vi "GSP_Wavelength_GenerateScript.vi"(0 "Current Grating":dbl, 1 "Current Camera":dbl, 2 "Target Grating":dbl, 3 "Target Camera":dbl, 4 "Move type":T1 items=["Both", "Grating Only", "Camera Only"]) -> (5 "Script":cluster{string, string}[](array[cluster]), 6 "AllowMove?":bool)   [LabVIEW 2015]
uses:
  movetypes.ctl
  wavelength_parameters.ctl
  GSCS Scripting/Utils/GSP_Wavelength_Global.vi
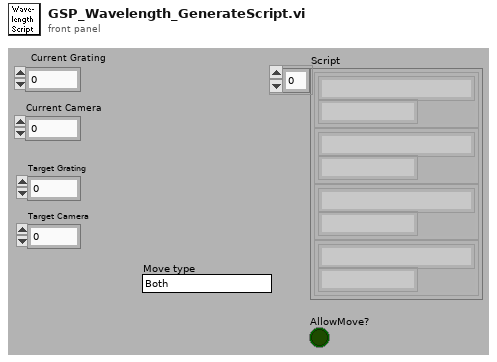
[diagram p1: front panel]
types:
  T1 = typedef "movetypes.ctl" = u16
  T2 = typedef "wavelength_parameters.ctl" = cluster{"Camera Angle":dbl, "Grating  Angle":dbl, "Move type":T1}
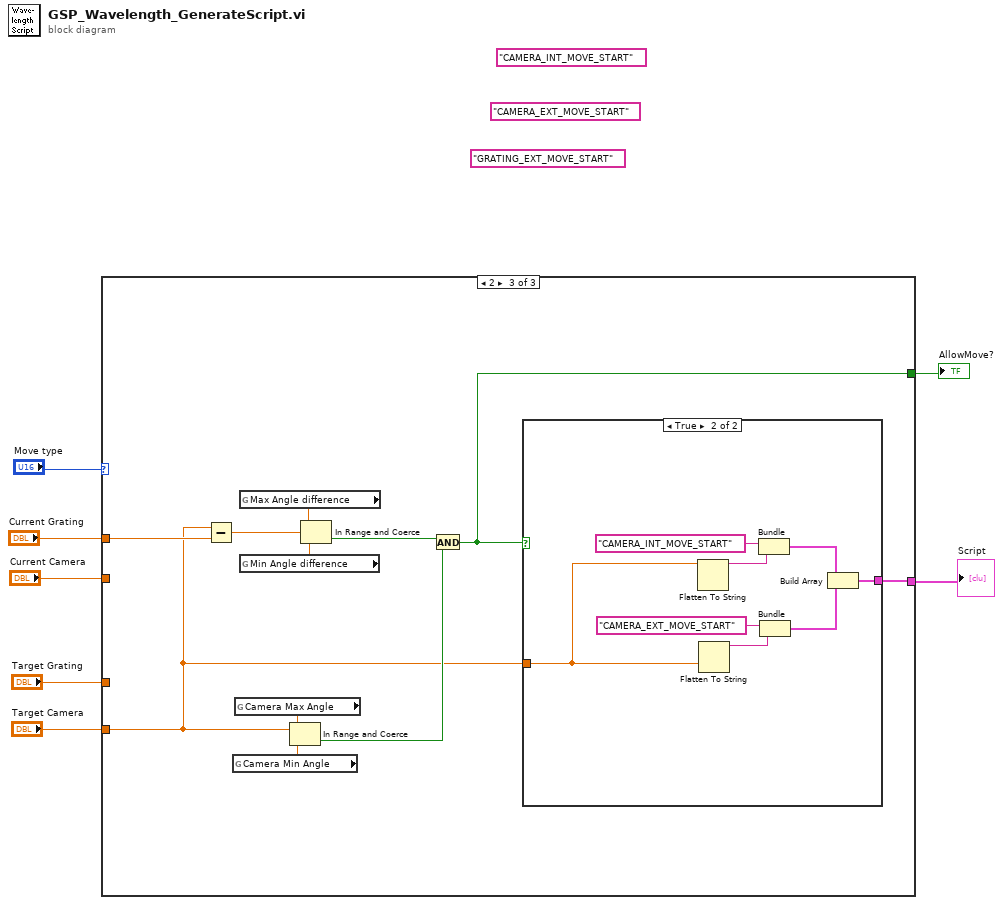
[diagram p0: block diagram]
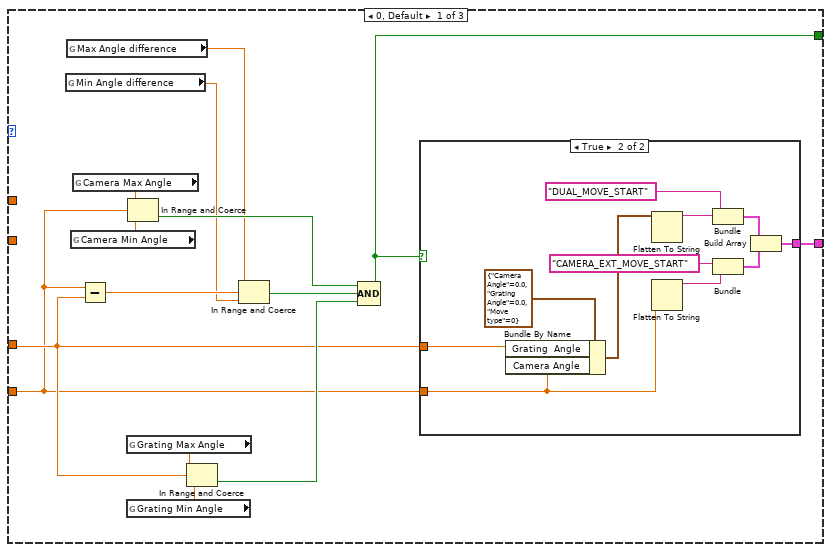
[diagram p2: hidden frame]
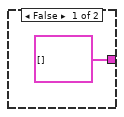
[diagram p3: hidden frame]
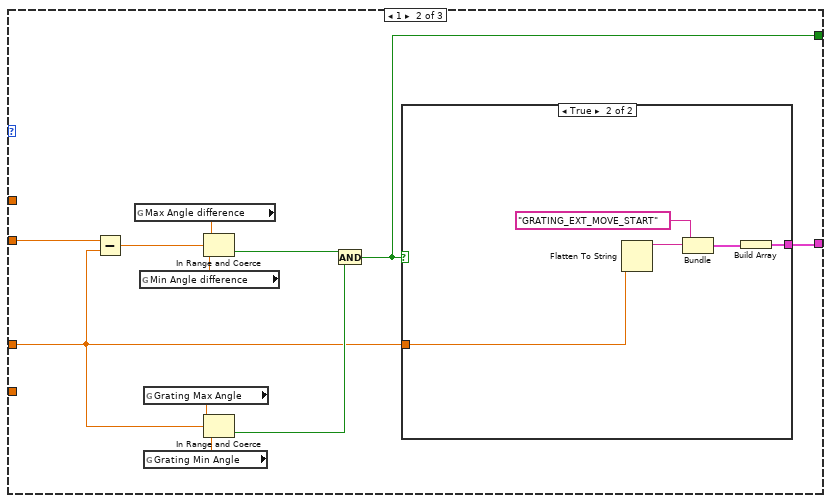
[diagram p4: hidden frame]
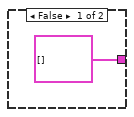
[diagram p5: hidden frame]
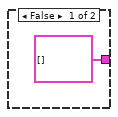
[diagram p6: hidden frame]
diagram:
  (unwired) "CAMERA_INT_MOVE_START"
  (unwired) "CAMERA_EXT_MOVE_START"
  (unwired) "GRATING_EXT_MOVE_START"
  n1 = case shown="2" "Move type" {
    tunnel: [w11 w34 w53] -> w6
    tunnel: "Current Grating" -> [_ _ w59]
    tunnel: "Current Camera" -> [_ w42 _]
    tunnel: "Target Grating" -> [w10 w35 _]
    tunnel: "Target Camera" -> [w9 _ w52]
    tunnel: [w8 w38 w51] -> w1
    frame 0, Default {
      n2 = global read "GSP_Wavelength_Global.vi" "Min Angle difference"() -> (w16:dbl)
      n3 = global read "GSP_Wavelength_Global.vi" "Max Angle difference"() -> (w17:dbl)
      n4 = global read "GSP_Wavelength_Global.vi" "Camera Min Angle"() -> (w14:dbl)
      n5 = global read "GSP_Wavelength_Global.vi" "Camera Max Angle"() -> (w15:dbl)
      n6 = Subtract(x=w9, y=w10) -> (x-y=w21:dbl)
      n7 = global read "GSP_Wavelength_Global.vi" "Grating Max Angle"() -> (w12:dbl)
      n8 = global read "GSP_Wavelength_Global.vi" "Grating Min Angle"() -> (w13:dbl)
      n9 = In Range and Coerce(upper limit=w15, x=w9, lower limit=w14) -> (In Range?=w19:bool)  [unwired: 1 out]
      n10 = In Range and Coerce(upper limit=w12, x=w10, lower limit=w13) -> (In Range?=w18:bool)  [unwired: 1 out]
      n11 = In Range and Coerce(upper limit=w17, x=w21, lower limit=w16) -> (In Range?=w20:bool)  [unwired: 1 out]
      n12 = Compound Arithmetic op=AND(w19, w20, w18) -> (w11:bool)
      n13 = case shown="True" w11 {
        tunnel: w10 -> [_ w32]
        tunnel: w9 -> [_ w27]
        tunnel: [cluster{string, "data string":string}[] [] w23] -> w8
        frame False {
        }
        frame True {
          n14 = Bundle By Name(cluster=T2 {"Camera Angle"=0.0, "Grating  Angle"=0.0, "Move type"=0} ("Wavelength Parameters"), "Grating  Angle"=w32, "Camera Angle"=w27) -> (w31:T2)
          n15 = Flatten To String(anything=w31) -> (data string=w29:string)  [unwired: 3 in, 2 out]
          n16 = Flatten To String(anything=w27) -> (data string=w26:string)  [unwired: 3 in, 2 out]
          n17 = Bundle("DUAL_MOVE_START", "data string"=w29) -> (w25:cluster{string, "data string":string})  [unwired: 1 in]
          n18 = Bundle("CAMERA_EXT_MOVE_START", "data string"=w26) -> (w24:cluster{string, "data string":string})  [unwired: 1 in]
          n19 = Build Array(w25, w24) -> (w23:cluster{string, "data string":string}[])
        }
      }
    }
    frame 1 {
      n20 = Subtract(x=w42, y=w35) -> (x-y=w41:dbl)
      n21 = global read "GSP_Wavelength_Global.vi" "Max Angle difference"() -> (w40:dbl)
      n22 = global read "GSP_Wavelength_Global.vi" "Min Angle difference"() -> (w39:dbl)
      n23 = global read "GSP_Wavelength_Global.vi" "Grating Max Angle"() -> (w43:dbl)
      n24 = global read "GSP_Wavelength_Global.vi" "Grating Min Angle"() -> (w44:dbl)
      n25 = In Range and Coerce(upper limit=w40, x=w41, lower limit=w39) -> (In Range?=w37:bool)  [unwired: 1 out]
      n26 = In Range and Coerce(upper limit=w43, x=w35, lower limit=w44) -> (In Range?=w36:bool)  [unwired: 1 out]
      n27 = And(x=w37, y=w36) -> (x .and. y?=w34:bool)
      n28 = case shown="True" w34 {
        tunnel: [cluster{string, "data string":string}[] [] w47] -> w38
        tunnel: w35 -> [_ w46]
        frame False {
        }
        frame True {
          n29 = Flatten To String(anything=w46) -> (data string=w49:string)  [unwired: 3 in, 2 out]
          n30 = Bundle("GRATING_EXT_MOVE_START", "data string"=w49) -> (w48:cluster{string, "data string":string})  [unwired: 1 in]
          n31 = Build Array(w48) -> (w47:cluster{string, "data string":string}[])
        }
      }
    }
    frame 2 {
      n32 = Subtract(x=w52, y=w59) -> (x-y=w56:dbl)
      n33 = global read "GSP_Wavelength_Global.vi" "Camera Min Angle"() -> (w60:dbl)
      n34 = global read "GSP_Wavelength_Global.vi" "Camera Max Angle"() -> (w61:dbl)
      n35 = global read "GSP_Wavelength_Global.vi" "Max Angle difference"() -> (w58:dbl)
      n36 = global read "GSP_Wavelength_Global.vi" "Min Angle difference"() -> (w57:dbl)
      n37 = In Range and Coerce(upper limit=w61, x=w52, lower limit=w60) -> (In Range?=w54:bool)  [unwired: 1 out]
      n38 = In Range and Coerce(upper limit=w58, x=w56, lower limit=w57) -> (In Range?=w55:bool)  [unwired: 1 out]
      n39 = And(x=w55, y=w54) -> (x .and. y?=w53:bool)
      n40 = case shown="True" w53 {
        tunnel: w52 -> [_ w64]
        tunnel: [cluster{string, "data string":string}[] [] w63] -> w51
        frame False {
        }
        frame True {
          n41 = Flatten To String(anything=w64) -> (data string=w67:string)  [unwired: 3 in, 2 out]
          n42 = Flatten To String(anything=w64) -> (data string=w69:string)  [unwired: 3 in, 2 out]
          n43 = Bundle("CAMERA_INT_MOVE_START", "data string"=w67) -> (w65:cluster{string, "data string":string})  [unwired: 1 in]
          n44 = Bundle("CAMERA_EXT_MOVE_START", "data string"=w69) -> (w66:cluster{string, "data string":string})  [unwired: 1 in]
          n45 = Build Array(w65, w66) -> (w63:cluster{string, "data string":string}[])
        }
      }
    }
  }
  "AllowMove?" <- w6
  "Script" <- w1
